vi "glob_var.vi"() -> ()   [LabVIEW 2010]
panel:
  in  "stop":bool caption="Stoppt alle Prozesse"
  in  "log_msg":string
  in  "new_log":bool
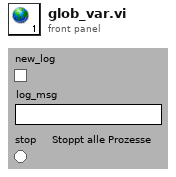
[diagram p1: front panel]
diagram:
